vi "SubVI_LR_Dashboard.vi"() -> (1 "First Char":string, 2 "Boolean":bool=TRUE)   [LabVIEW 2017]
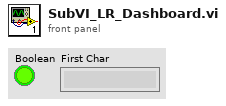
[diagram p1: front panel]
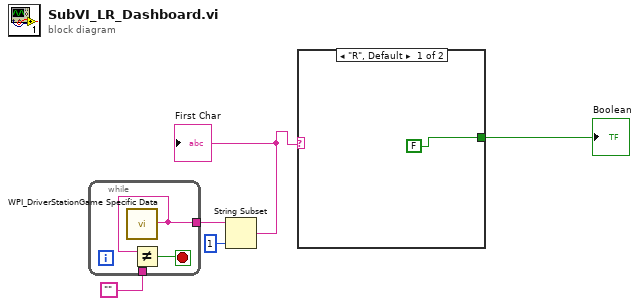
[diagram p0: block diagram]
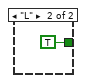
[diagram p2: hidden frame]
diagram:
  n1 = while {
    tunnel: [w7] -> w5
    tunnel: "" -> [w8]
    stop <- w6 stop-if-true
    n2 = call <vilib>:"WPI_DriverStationGame Specific Data.vi"() -> ("Game Specific Data"=w7:string)  [unwired: 11 in]
    n3 = Not Equal?(x=w7, y=w8) -> (x != y?=w6:bool)
  }
  n4 = String Subset(string=w5, length (rest)=1 ("length (rest)")) -> (substring=w3:string)  [unwired: 1 in]
  "First Char" <- w3
  n5 = case shown="\"R\", Default" w3 {
    tunnel: [FALSE TRUE] -> w2
    frame "R", Default {
    }
    frame "L" {
    }
  }
  "Boolean" <- w2
